vi "Main.vi"(8 "DB-Interface":refnum<class "DB-Interface.lvclass">, 9 "Call Chain":string[](array[string]), 10 "Config Section":string, 11 "Module Admin":refnum<class "Delacor_lib_QMH_Cloneable Module Admin.lvclass">) -> ()   [LabVIEW 2022 SP3, in "hse-db.lvlib" / "DB_CONNECTOR.lvlib"]
doc: "Database Connector DQMH module. \n\nThis module is a singleton. Every module or component within an application that needs database connectivity should load its own instance of this module and keep the reference private.\n\n____\nHAMPEL SOFTWARE ENGINEERING v1.4.0 (2023-12-19 09:52)"
uses:
  DB_CONNECTOR.lvlib
  <vilib>/Delacor/Delacor QMH/Libraries/Cloneable Module Admin_class/Delacor_lib_QMH_Cloneable Module Admin.lvclass
  C:/Program Files/National Instruments/LabVIEW 2022/vi.lib/Delacor/Delacor QMH/Libraries/Module Admin_class/Delacor_lib_QMH_Module Admin.lvclass
  DB-Interface/DB-Interface.lvclass
  Module Data--cluster.ctl
  hse-libraries/Source/hse-configuration/config-base/config-base.lvclass
  Stop Argument--cluster.ctl
  <vilib>/Delacor/Delacor QMH/Libraries/Message Queue_class/Delacor_lib_QMH_Message Queue.lvclass/Delacor_lib_QMH_Message Queue.ctl
  <vilib>/Delacor/Delacor QMH/Libraries/Module Admin_class/Delacor_lib_QMH_Module Admin.lvclass/Delacor_lib_QMH_Module Admin.ctl
  <vilib>/Delacor/Delacor QMH/Libraries/Cloneable Module Admin_class/Delacor_lib_QMH_Cloneable Module Admin.lvclass/Delacor_lib_QMH_Cloneable Module Admin.ctl
  Configure Argument--cluster.ctl
  Connect Argument--cluster.ctl
  Fast Query Argument--cluster.ctl
  Close Connection Argument--cluster.ctl
  Start Transaction Argument--cluster.ctl
  Get DB-Type Argument--cluster.ctl
  Get DB-Type (Reply Payload)--cluster.ctl
  Query Argument--cluster.ctl
  Query (Reply Payload)--cluster.ctl
  Commit Transaction Argument--cluster.ctl
  Commit Transaction (Reply Payload)--cluster.ctl
  Set Module Timeout Argument--cluster.ctl
  Rollback Transaction Argument--cluster.ctl
  Rollback Transaction (Reply Payload)--cluster.ctl
  Sub-VIs/timeout-fgv-actions--control.ctl
  <vilib>/Utility/miscctls.llb/LVPointTypeDef.ctl
  <vilib>/Delacor/Delacor QMH/Libraries/Message Queue_class/Delacor_lib_QMH_Enqueue Message (Single).vi
  <vilib>/Delacor/Delacor QMH/Libraries/Cloneable Module Admin_class/Delacor_lib_QMH_Get Module ID.vi
  <vilib>/Delacor/Delacor QMH/Libraries/Module Admin_class/Delacor_lib_QMH_Get External Launch.vi
  <vilib>/Utility/error.llb/Error Cluster From Error Code.vi
  <vilib>/ErrorRing/Error Ring.xnode
  <vilib>/Delacor/Delacor QMH/Libraries/Message Queue_class/Delacor_lib_QMH_Message Queue.lvclass
panel:
  out "Module Name":string
  out "error out":errorcluster
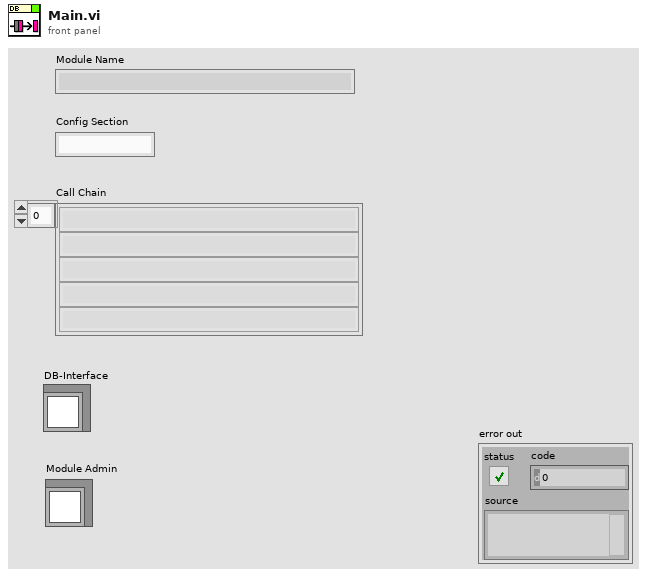
[diagram p1: front panel]
types:
  T1 = typedef "hse-db.lvlib/DB_CONNECTOR.lvlib/Request Events--cluster.ctl" = cluster{"Stop Module":refnum<user-event>, "Show Panel":refnum<user-event>, "Hide Panel":refnum<user-event>, "Show Diagram":refnum<user-event>, "Get Module Execution Status":refnum<user-event>, "Configure":refnum<user-event>, "Connect":refnum<user-event>, "Close Connection":refnum<user-event>, "Start Transaction":refnum<user-event>, "Fast Query":refnum<user-event>, "Get DB-Type":refnum<user-event>, "Query":refnum<user-event>, "Commit Transaction":refnum<user-event>, "Set Module Timeout":refnum<user-event>, "Rollback Transaction":refnum<user-event>}
  T2 = typedef "hse-db.lvlib/DB_CONNECTOR.lvlib/Module Data--cluster.ctl" = cluster{"hse-config":refnum<class "config-base.lvclass">, "Config Section":string, "DB-Interface":refnum<class "DB-Interface.lvclass">}
  T3 = enum32{"invalid lock state", "Not Locked", "Locked (No Password)", "Password-protected"}
  T4 = typedef "hse-db.lvlib/DB_CONNECTOR.lvlib/Stop Argument--cluster.ctl" = cluster{"Origin":string, "Module ID":i32, "Exit via Stop Module Req?":bool, "Wait for Module to stop?":bool}
  T5 = typedef "hse-db.lvlib/DB_CONNECTOR.lvlib/Configure Argument--cluster.ctl" = cluster{"Module ID":i32, "Boolean":bool}
  T6 = typedef "hse-db.lvlib/DB_CONNECTOR.lvlib/Connect Argument--cluster.ctl" = cluster{"Module ID":i32, "Boolean":bool}
  T7 = typedef "hse-db.lvlib/DB_CONNECTOR.lvlib/Fast Query Argument--cluster.ctl" = cluster{"Module ID":i32, "Query":string}
  T8 = typedef "hse-db.lvlib/DB_CONNECTOR.lvlib/Close Connection Argument--cluster.ctl" = cluster{"Module ID":i32, "Boolean":bool}
  T9 = typedef "hse-db.lvlib/DB_CONNECTOR.lvlib/Start Transaction Argument--cluster.ctl" = cluster{"Module ID":i32, "Boolean":bool}
  T10 = typedef "hse-db.lvlib/DB_CONNECTOR.lvlib/Get DB-Type Argument--cluster.ctl" = cluster{"Module ID":i32, "Wait Notifier":refnum<notifier>, "wait for reply":bool}
  T11 = typedef "hse-db.lvlib/DB_CONNECTOR.lvlib/Query Argument--cluster.ctl" = cluster{"Module ID":i32, "Query":string, "Wait Notifier":refnum<notifier>, "wait for reply":bool}
  T12 = typedef "hse-db.lvlib/DB_CONNECTOR.lvlib/Commit Transaction Argument--cluster.ctl" = cluster{"Module ID":i32, "Wait Notifier":refnum<notifier>, "wait for reply":bool}
  T13 = typedef "hse-db.lvlib/DB_CONNECTOR.lvlib/Set Module Timeout Argument--cluster.ctl" = cluster{"Module ID":i32, "Module Timeout":i32}
  T14 = typedef "hse-db.lvlib/DB_CONNECTOR.lvlib/Rollback Transaction Argument--cluster.ctl" = cluster{"Module ID":i32, "Wait Notifier":refnum<notifier>, "wait for reply":bool}
  T15 = typedef "hse-db.lvlib/DB_CONNECTOR.lvlib/timeout-fgv-actions--control.ctl" = enum16{"set", "get"}
  T16 = typedef "LVPointTypeDef.ctl" = cluster{"Horizontal":i16, "Vertical":i16}
  T17 = enum32{"Invalid", "Standard", "Closed", "Hidden", "Minimized", "Maximized"}
  T18 = typedef "hse-db.lvlib/DB_CONNECTOR.lvlib/Query (Reply Payload)--cluster.ctl" = cluster{"Return Data":string[][], "Meta Data":variant, "Field Names":string[], "Query_error":errorcluster, "Module ID":i32}
  T19 = typedef "hse-db.lvlib/DB_CONNECTOR.lvlib/Commit Transaction (Reply Payload)--cluster.ctl" = cluster{"Commit Transaction_error":errorcluster, "Module ID":i32}
  T20 = typedef "hse-db.lvlib/DB_CONNECTOR.lvlib/Rollback Transaction (Reply Payload)--cluster.ctl" = cluster{"Rollback Transaction_error":errorcluster, "Module ID":i32}
  T21 = typedef "hse-db.lvlib/DB_CONNECTOR.lvlib/Get DB-Type (Reply Payload)--cluster.ctl" = cluster{"DB-Type":string, "error":errorcluster, "Module ID":i32}
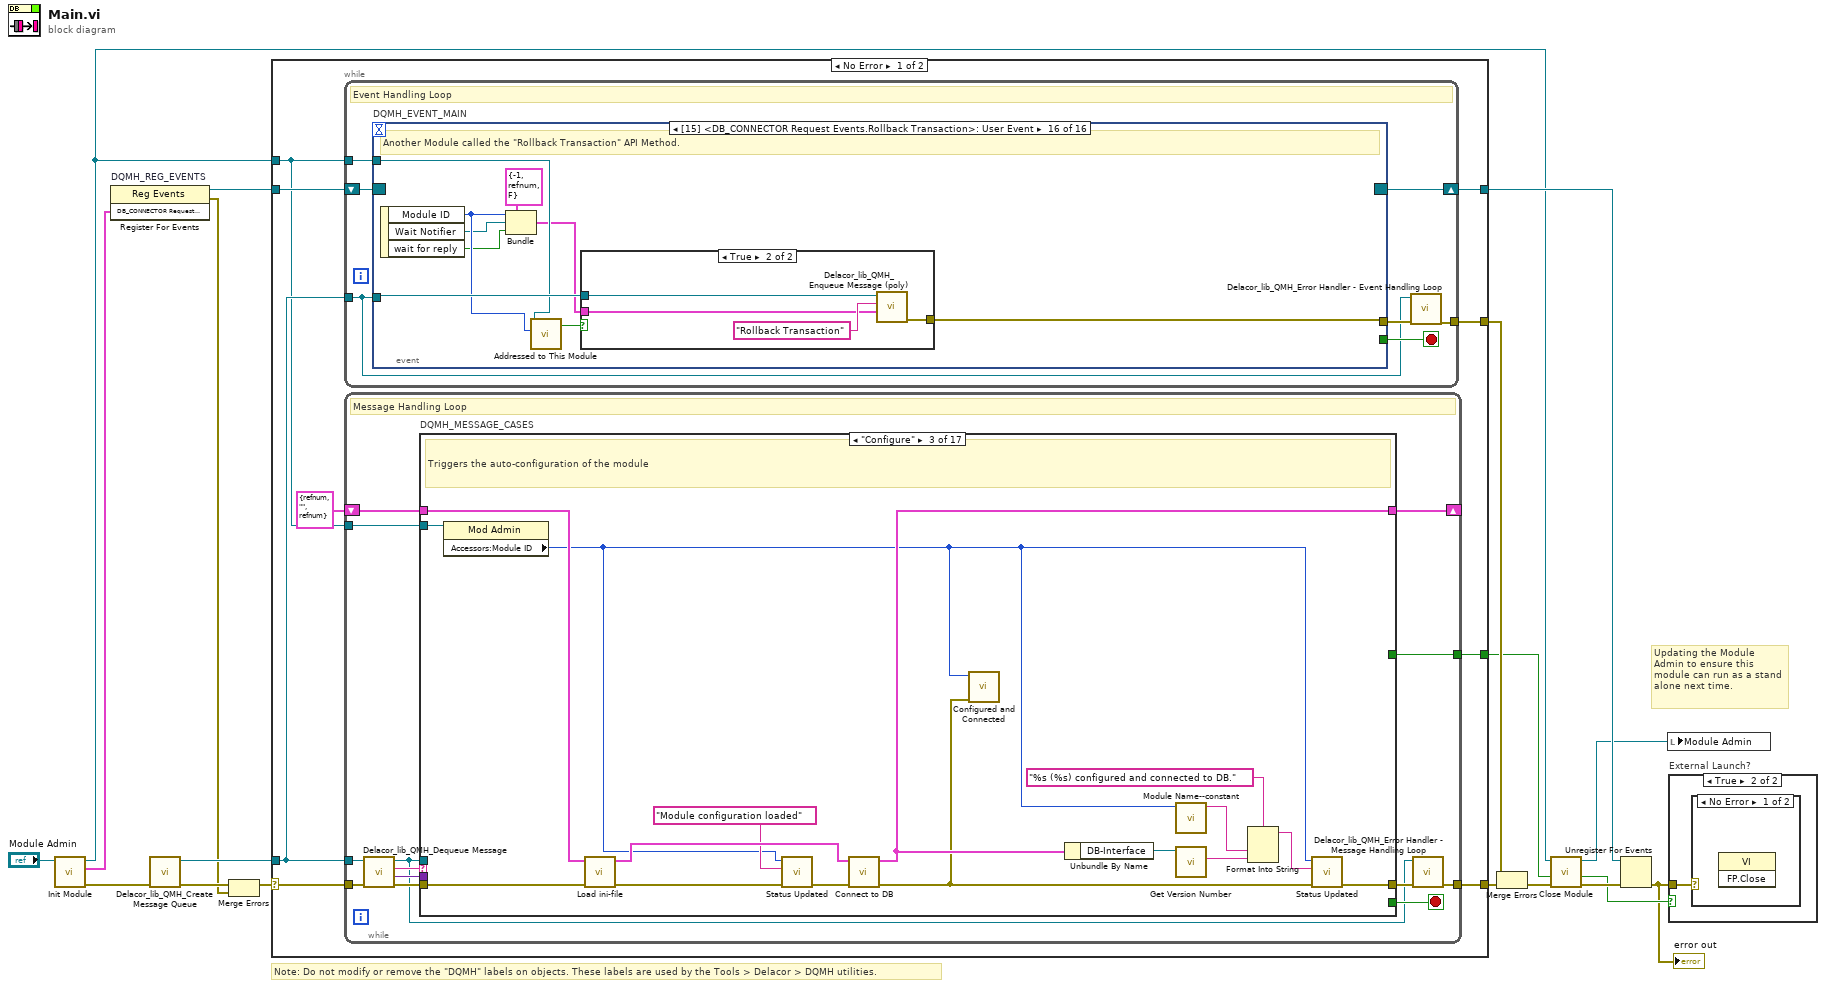
[diagram p0: block diagram]
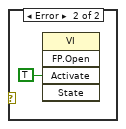
[diagram p3: hidden frame]
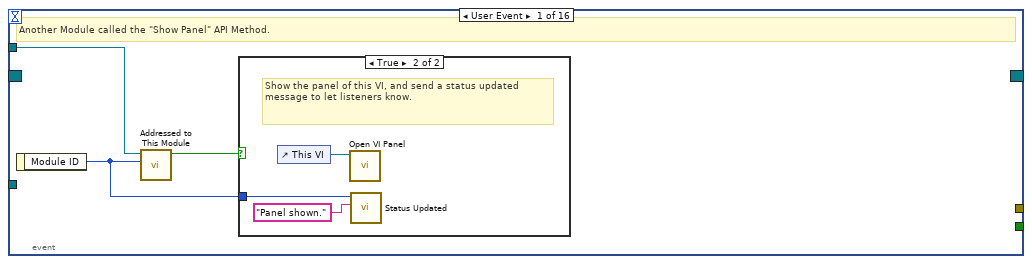
[diagram p4: hidden frame]
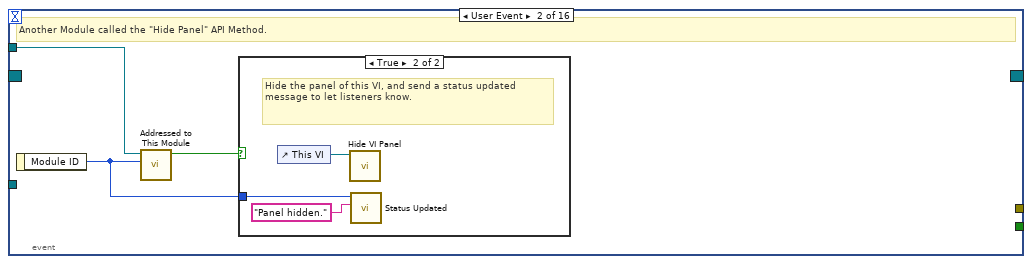
[diagram p6: hidden frame]
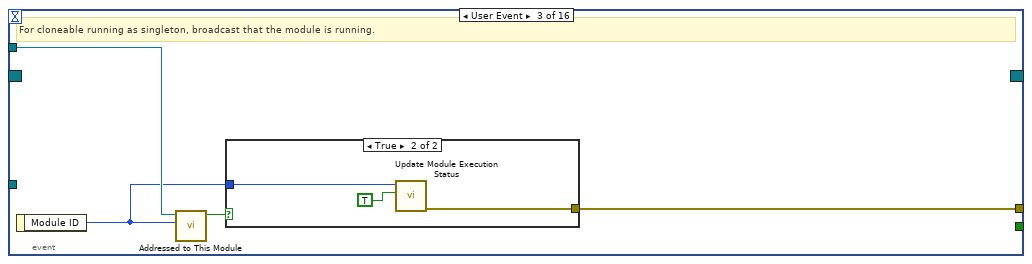
[diagram p8: hidden frame]
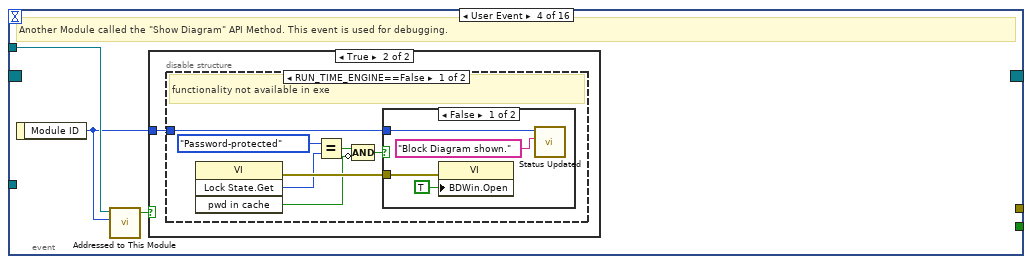
[diagram p10: hidden frame]
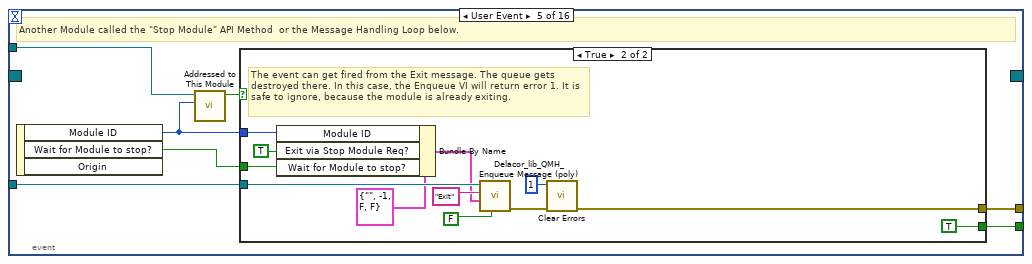
[diagram p14: hidden frame]
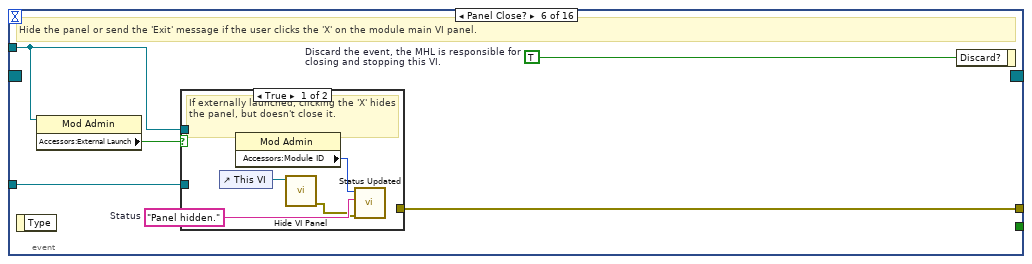
[diagram p16: hidden frame]
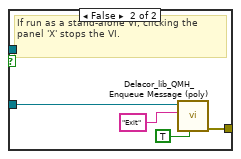
[diagram p17: hidden frame]
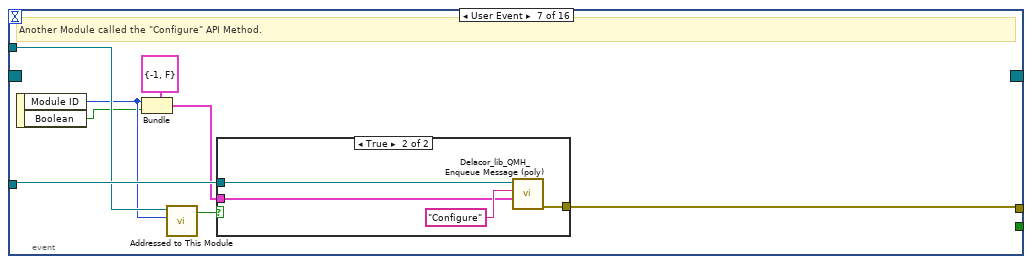
[diagram p18: hidden frame]
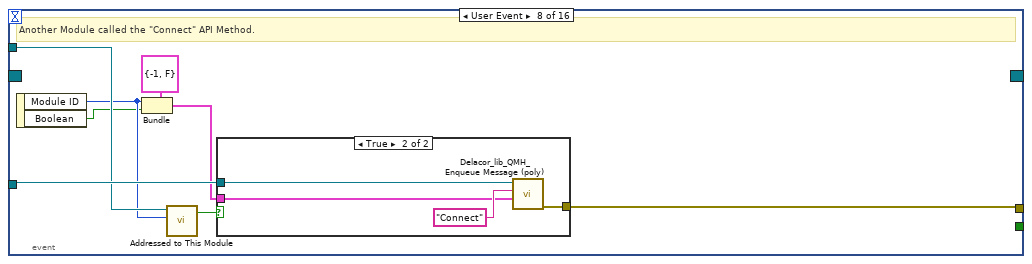
[diagram p20: hidden frame]
diagram:
  # "Note: Do not modify or remove the \"DQMH\" labels on objects. These labels are used by the Tools > Delacor > DQMH utilities."
  # "Updating the Module Admin to ensure this module can run as a stand alone next time."
  n1 = call "Init Module.vi"("Cloneable Module Admin in"="Module Admin") -> ("error out"=w15:errorcluster, "DB_CONNECTOR Request Events"=w12:T1, "Cloneable Module Admin out"=w8:refnum<class "Delacor_lib_QMH_Cloneable Module Admin.lvclass">)  [unwired: 8 in]
  n2 = register-events "DQMH_REG_EVENTS"(w12) -> (reference out=w13:refnum<event-registration>, error out=w3:errorcluster)  [unwired: 2 in]
  n3 = call <vilib>:"Delacor_lib_QMH_Create Message Queue.vi"("error in"=w15) -> ("error out"=w5:errorcluster, "Message Queue"=w11:refnum<class "Delacor_lib_QMH_Message Queue.lvclass">)  [unwired: 9 in]
  n4 = Merge Errors(w5, w3) -> (w4:errorcluster)
  n5 = case shown="No Error" w4 {
    selector: w4 -> [w21 w514]
    tunnel: [w27 w514] -> w16
    tunnel: [w26 w515] -> w14
    tunnel: w13 -> [w24 w515]
    tunnel: w11 -> [w23 w507]
    tunnel: [w22 _] -> w17
    tunnel: w8 -> [w20 w510]
    tunnel: [w19 _] -> w7
    frame No Error {
      n6 = while {
        tunnel: w23 -> [w28]
        shift-right: [w33] -> w26
        shift-left: w24 -> [w34]
        tunnel: [w30] -> w22
        tunnel: w20 -> [w29]
        stop <- w31 stop-if-true
        # "Event Handling Loop"
        n7 = event "DQMH_EVENT_MAIN" shown="[15] <DB_CONNECTOR Request Events.Rollback Transaction>: User Event" {
          selector: w34 -> [_ _ _ _ _ _ _ _ _ _ _ _ _ _ _ _]
          dyn-events: [_ _ _ _ _ _ _ _ _ _ _ _ _ _ _ _] -> w33
          timeout: _ -> [_ _ _ _ _ _ _ _ _ _ _ _ _ _ _ _]
          tunnel: [_ _ _ _ w72 _ _ _ _ _ _ _ _ _ _ _] -> w31
          tunnel: w28 -> [_ _ _ _ w75 w91 w109 w121 w133 w145 w157 w170 w184 w197 w209 w222]
          tunnel: [_ _ w48 _ w69 w89 w102 w114 w126 w138 w150 w162 w179 w192 w202 w214] -> w32
          tunnel: w29 -> [w36 w42 w49 w55 w74 w88 w107 w119 w131 w143 w155 w168 w182 w195 w207 w220]
          event User Event {
            # "Another Module called the \"Show Panel\" API Method."
            n8 = event-data() -> ("Module ID"=w35:i32)  [unwired: 1 in]
            n9 = call "Addressed to This Module.vi"("Module ID from Argument"=w35, "Module Admin"=w36) -> ("Addressed to this instance?"=w37:bool)  [unwired: 8 in, 1 out]
            n10 = case shown="True" w37 {
              tunnel: w35 -> [_ w38]
              frame False {
              }
              frame True {
                # "Show the panel of this VI, and send a status updated message to let listeners know."
                n11 = control-ref of="This VI"() -> (w40:refnum<vi>)
                n12 = call "Open VI Panel.vi"("VI"=w40) -> ()  [unwired: 10 in, 1 out]
                n13 = call "Status Updated.vi"("Status"="Panel shown." ("format string"), "Module ID"=w38) -> ()  [unwired: 9 in, 1 out]
              }
            }
          }
          event User Event {
            # "Another Module called the \"Hide Panel\" API Method."
            n14 = event-data() -> ("Module ID"=w41:i32)  [unwired: 1 in]
            n15 = call "Addressed to This Module.vi"("Module ID from Argument"=w41, "Module Admin"=w42) -> ("Addressed to this instance?"=w43:bool)  [unwired: 8 in, 1 out]
            n16 = case shown="True" w43 {
              tunnel: w41 -> [_ w44]
              frame False {
              }
              frame True {
                # "Hide the panel of this VI, and send a status updated message to let listeners know."
                n17 = control-ref of="This VI"() -> (w46:refnum<vi>)
                n18 = call "Hide VI Panel.vi"("VI"=w46) -> ()  [unwired: 10 in, 1 out]
                n19 = call "Status Updated.vi"("Status"="Panel hidden." ("format string"), "Module ID"=w44) -> ()  [unwired: 9 in, 1 out]
              }
            }
          }
          event User Event {
            # "For cloneable running as singleton, broadcast that the module is running."
            n20 = event-data() -> ("Module ID"=w47:i32)  [unwired: 1 in]
            n21 = call "Addressed to This Module.vi"("Module ID from Argument"=w47, "Module Admin"=w49) -> ("Addressed to this instance?"=w50:bool)  [unwired: 8 in, 1 out]
            n22 = case shown="True" w50 {
              tunnel: [_ w53] -> w48
              tunnel: w47 -> [_ w52]
              frame False {
              }
              frame True {
                n23 = call "Update Module Execution Status.vi"("Running?"=TRUE, "Module ID"=w52) -> ("error out"=w53:errorcluster)  [unwired: 9 in]
              }
            }
          }
          event User Event {
            # "Another Module called the \"Show Diagram\" API Method. This event is used for debugging."
            n24 = event-data() -> ("Module ID"=w54:i32)  [unwired: 1 in]
            n25 = call "Addressed to This Module.vi"("Module ID from Argument"=w54, "Module Admin"=w55) -> ("Addressed to this instance?"=w56:bool)  [unwired: 8 in, 1 out]
            n26 = case shown="True" w56 {
              tunnel: w54 -> [_ w57]
              frame False {
              }
              frame True {
                n27 = disable-structure shown="RUN_TIME_ENGINE==False" {
                  disable-tunnel: w57 -> [w58 _]
                  frame condition #0 (active) {
                    # "functionality not available in exe"
                    n28 = invoke on="Invoke Node" class="VI" method="Lock State.Get"() -> (error out=w64:errorcluster, "Get Lock State"=w63:T3, "pwd in cache"=w60:bool)  [unwired: 4 in, 1 out]
                    n29 = Equal?(x=T3."Password-protected", y=w63) -> (x = y?=w61:bool)
                    n30 = Compound Arithmetic op=AND(w61, invert w60) -> (w59:bool)
                    n31 = case shown="False" w59 {
                      tunnel: w64 -> [w67 _]
                      tunnel: w58 -> [w65 _]
                      frame False {
                        n32 = property on="Property Node" class="VI"(error in=w67, "BDWin.Open"=TRUE ("Block Diagram Window:Open")) -> ()  [unwired: 1 in, 2 out]
                        n33 = call "Status Updated.vi"("Status"="Block Diagram shown." ("format string"), "Module ID"=w65) -> ()  [unwired: 9 in, 1 out]
                      }
                      frame True {
                        # "Password-protected VI, and the password is not in the cache. Do not show the diagram."
                      }
                    }
                  }
                  frame condition #1 {
                  }
                }
              }
            }
          }
          event User Event {
            # "Another Module called the \"Stop Module\" API Method  or the Message Handling Loop below."
            n34 = event-data() -> ("Module ID"=w70:i32, "Wait for Module to stop?"=w71:bool)  [unwired: 1 in, 1 out]
            n35 = call "Addressed to This Module.vi"("Module ID from Argument"=w70, "Module Admin"=w74) -> ("Addressed to this instance?"=w73:bool)  [unwired: 8 in, 1 out]
            n36 = case shown="True" w73 {
              tunnel: [_ w77] -> w69
              tunnel: w75 -> [_ w83]
              tunnel: [_ TRUE] -> w72
              tunnel: w71 -> [_ w79]
              tunnel: w70 -> [_ w76]
              frame False {
              }
              frame True {
                # "The event can get fired from the Exit message. The queue gets destroyed there. In this case, the Enqueue VI will return error 1. It is safe to ignore, because the module is already exiting."
                n37 = Bundle By Name(cluster=T4 {"Origin"="", "Module ID"=-1, "Exit via Stop Module Req?"=FALSE, "Wait for Module to stop?"=FALSE} ("Stop Argument"), "Module ID"=w76, "Exit via Stop Module Req?"=TRUE, "Wait for Module to stop?"=w79) -> (w78:T4)
                n38 = call-poly <vilib>:"Delacor_lib_QMH_Enqueue Message (poly).vi"("Priority Message? (F)"=FALSE, "Message Data"=w78, "Message"="Exit", "Message Queue in"=w83) -> ("error out"=w86:errorcluster)  [unwired: 6 in, 1 out]
                n39 = call <vilib>:"Clear Errors.vi"("error in (no error)"=w86, "specific error code to clear (0: all)"=1) -> ("error out"=w77:errorcluster)  [unwired: 4 in, 1 out]
              }
            }
          }
          event Panel Close? {
            w92 = TRUE  # Discard the event, the MHL is responsible for closing and stopping this VI.
            # "Hide the panel or send the 'Exit' message if the user clicks the 'X' on the module main VI panel."
            n40 = event-data() -> ()  [unwired: 1 in, 1 out]
            n41 = property on="Property Node" class="Mod Admin"(reference=w88) -> ("Accessors:External Launch"=w90:bool)  [unwired: 1 in, 2 out]
            n42 = case shown="True" w90 {
              tunnel: w91 -> [_ w101]
              tunnel: [_ w100] -> w89
              tunnel: w88 -> [w95 _]
              frame True {
                w96 = "Panel hidden."  # Status
                # "If externally launched, clicking the 'X' hides the panel, but doesn't close it."
                n43 = control-ref of="This VI"() -> (w97:refnum<vi>)
                n44 = property class="Mod Admin"(reference=w95) -> ("Accessors:Module ID"=w94:i32)  [unwired: 1 in, 2 out]
                n45 = call "Hide VI Panel.vi"("VI"=w97) -> ("error out"=w93:errorcluster)  [unwired: 10 in]
                n46 = call "Status Updated.vi"("error in (no error)"=w93, "Status"=w96, "Module ID"=w94) -> ()  [unwired: 8 in, 1 out]
              }
              frame False {
                # "If run as a stand-alone VI, clicking the panel 'X' stops the VI."
                n47 = call-poly <vilib>:"Delacor_lib_QMH_Enqueue Message (poly).vi"("Priority Message? (F)"=TRUE, "Message"="Exit", "Message Queue in"=w101) -> ("error out"=w100:errorcluster)  [unwired: 7 in, 1 out]
              }
            }
            n48 = event-data ("Event Filter Node")("Discard?"=w92) -> ()  [unwired: 1 in, 1 out]
          }
          event User Event {
            # "Another Module called the \"Configure\" API Method."
            n49 = event-data() -> ("Module ID"=w104:i32, "Boolean"=w103:bool)  [unwired: 1 in]
            n50 = Bundle(cluster=T5 {"Module ID"=-1, "Boolean"=FALSE} ("Configure Argument"), "Module ID"=w104, "Boolean"=w103) -> (w105:T5)
            n51 = call "Addressed to This Module.vi"("Module ID from Argument"=w104, "Module Admin"=w107) -> ("Addressed to this instance?"=w108:bool)  [unwired: 8 in, 1 out]
            n52 = case shown="True" w108 {
              tunnel: w109 -> [_ w113]
              tunnel: w105 -> [_ w111]
              tunnel: [_ w110] -> w102
              frame False {
              }
              frame True {
                n53 = call-poly <vilib>:"Delacor_lib_QMH_Enqueue Message (poly).vi"("Message Data"=w111, "Message"="Configure", "Message Queue in"=w113) -> ("error out"=w110:errorcluster)  [unwired: 7 in, 1 out]
              }
            }
          }
          event User Event {
            # "Another Module called the \"Connect\" API Method."
            n54 = event-data() -> ("Module ID"=w116:i32, "Boolean"=w115:bool)  [unwired: 1 in]
            n55 = Bundle(cluster=T6 {"Module ID"=-1, "Boolean"=FALSE} ("Connect Argument"), "Module ID"=w116, "Boolean"=w115) -> (w117:T6)
            n56 = call "Addressed to This Module.vi"("Module ID from Argument"=w116, "Module Admin"=w119) -> ("Addressed to this instance?"=w120:bool)  [unwired: 8 in, 1 out]
            n57 = case shown="True" w120 {
              tunnel: w121 -> [_ w125]
              tunnel: w117 -> [_ w123]
              tunnel: [_ w122] -> w114
              frame False {
              }
              frame True {
                n58 = call-poly <vilib>:"Delacor_lib_QMH_Enqueue Message (poly).vi"("Message Data"=w123, "Message"="Connect", "Message Queue in"=w125) -> ("error out"=w122:errorcluster)  [unwired: 7 in, 1 out]
              }
            }
          }
          event User Event {
            # "Another Module called the \"Fast Query\" API Method."
            n59 = event-data() -> ("Module ID"=w128:i32, "Query"=w127:string)  [unwired: 1 in]
            n60 = Bundle(cluster=T7 {"Module ID"=-1, "Query"=""} ("Fast Query Argument"), "Module ID"=w128, "Query"=w127) -> (w129:T7)
            n61 = call "Addressed to This Module.vi"("Module ID from Argument"=w128, "Module Admin"=w131) -> ("Addressed to this instance?"=w132:bool)  [unwired: 8 in, 1 out]
            n62 = case shown="True" w132 {
              tunnel: w133 -> [_ w137]
              tunnel: w129 -> [_ w135]
              tunnel: [_ w134] -> w126
              frame False {
              }
              frame True {
                n63 = call-poly <vilib>:"Delacor_lib_QMH_Enqueue Message (poly).vi"("Message Data"=w135, "Message"="Fast Query", "Message Queue in"=w137) -> ("error out"=w134:errorcluster)  [unwired: 7 in, 1 out]
              }
            }
          }
          event User Event {
            # "Another Module called the \"Close Connection\" API Method."
            n64 = event-data() -> ("Module ID"=w140:i32, "Boolean"=w139:bool)  [unwired: 1 in]
            n65 = Bundle(cluster=T8 {"Module ID"=-1, "Boolean"=FALSE} ("Close Connection Argument"), "Module ID"=w140, "Boolean"=w139) -> (w141:T8)
            n66 = call "Addressed to This Module.vi"("Module ID from Argument"=w140, "Module Admin"=w143) -> ("Addressed to this instance?"=w144:bool)  [unwired: 8 in, 1 out]
            n67 = case shown="True" w144 {
              tunnel: w145 -> [_ w149]
              tunnel: w141 -> [_ w147]
              tunnel: [_ w146] -> w138
              frame False {
              }
              frame True {
                n68 = call-poly <vilib>:"Delacor_lib_QMH_Enqueue Message (poly).vi"("Message Data"=w147, "Message"="Close Connection", "Message Queue in"=w149) -> ("error out"=w146:errorcluster)  [unwired: 7 in, 1 out]
              }
            }
          }
          event User Event {
            # "Another Module called the \"Start Transaction\" API Method."
            n69 = event-data() -> ("Module ID"=w152:i32, "Boolean"=w151:bool)  [unwired: 1 in]
            n70 = Bundle(cluster=T9 {"Module ID"=-1, "Boolean"=FALSE} ("Start Transaction Argument"), "Module ID"=w152, "Boolean"=w151) -> (w153:T9)
            n71 = call "Addressed to This Module.vi"("Module ID from Argument"=w152, "Module Admin"=w155) -> ("Addressed to this instance?"=w156:bool)  [unwired: 8 in, 1 out]
            n72 = case shown="True" w156 {
              tunnel: w157 -> [_ w161]
              tunnel: w153 -> [_ w159]
              tunnel: [_ w158] -> w150
              frame False {
              }
              frame True {
                n73 = call-poly <vilib>:"Delacor_lib_QMH_Enqueue Message (poly).vi"("Message Data"=w159, "Message"="Start Transaction", "Message Queue in"=w161) -> ("error out"=w158:errorcluster)  [unwired: 7 in, 1 out]
              }
            }
          }
          event User Event {
            # "Another Module called the \"Get DB-Type\" API Method."
            n74 = event-data() -> ("Module ID"=w165:i32, "Wait Notifier"=w164:refnum<notifier>, "wait for reply"=w163:bool)  [unwired: 1 in]
            n75 = Bundle(cluster=T10 {"Module ID"=-1, "Wait Notifier"=refnum, "wait for reply"=FALSE} ("Get DB-Type Argument"), "Module ID"=w165, "Wait Notifier"=w164, "wait for reply"=w163) -> (w166:T10)
            n76 = call "Addressed to This Module.vi"("Module ID from Argument"=w165, "Module Admin"=w168) -> ("Addressed to this instance?"=w169:bool)  [unwired: 8 in, 1 out]
            n77 = case shown="True" w169 {
              tunnel: w170 -> [_ w174]
              tunnel: w166 -> [_ w172]
              tunnel: [_ w171] -> w162
              frame False {
              }
              frame True {
                n78 = call-poly <vilib>:"Delacor_lib_QMH_Enqueue Message (poly).vi"("Message Data"=w172, "Message"="Get DB-Type", "Message Queue in"=w174) -> ("error out"=w171:errorcluster)  [unwired: 7 in, 1 out]
              }
            }
          }
          event User Event {
            # "Another Module called the \"Query\" API Method."
            n79 = event-data() -> ("Module ID"=w175:i32, "Query"=w178:string, "Wait Notifier"=w177:refnum<notifier>, "wait for reply"=w176:bool)  [unwired: 1 in]
            n80 = Bundle(cluster=T11 {"Module ID"=-1, "Query"="", "Wait Notifier"=refnum, "wait for reply"=FALSE} ("Query Argument"), "Module ID"=w175, "Query"=w178, "Wait Notifier"=w177, "wait for reply"=w176) -> (w180:T11)
            n81 = call "Addressed to This Module.vi"("Module ID from Argument"=w175, "Module Admin"=w182) -> ("Addressed to this instance?"=w183:bool)  [unwired: 8 in, 1 out]
            n82 = case shown="True" w183 {
              tunnel: w184 -> [_ w188]
              tunnel: w180 -> [_ w186]
              tunnel: [_ w185] -> w179
              frame False {
              }
              frame True {
                n83 = call-poly <vilib>:"Delacor_lib_QMH_Enqueue Message (poly).vi"("Message Data"=w186, "Message"="Query", "Message Queue in"=w188) -> ("error out"=w185:errorcluster)  [unwired: 7 in, 1 out]
              }
            }
          }
          event User Event {
            # "Another Module called the \"Commit Transaction\" API Method."
            n84 = event-data() -> ("Module ID"=w189:i32, "Wait Notifier"=w191:refnum<notifier>, "wait for reply"=w190:bool)  [unwired: 1 in]
            n85 = Bundle(cluster=T12 {"Module ID"=-1, "Wait Notifier"=refnum, "wait for reply"=FALSE} ("Commit Transaction Argument"), "Module ID"=w189, "Wait Notifier"=w191, "wait for reply"=w190) -> (w193:T12)
            n86 = call "Addressed to This Module.vi"("Module ID from Argument"=w189, "Module Admin"=w195) -> ("Addressed to this instance?"=w196:bool)  [unwired: 8 in, 1 out]
            n87 = case shown="True" w196 {
              tunnel: w197 -> [_ w201]
              tunnel: w193 -> [_ w199]
              tunnel: [_ w198] -> w192
              frame False {
              }
              frame True {
                n88 = call-poly <vilib>:"Delacor_lib_QMH_Enqueue Message (poly).vi"("Message Data"=w199, "Message"="Commit Transaction", "Message Queue in"=w201) -> ("error out"=w198:errorcluster)  [unwired: 7 in, 1 out]
              }
            }
          }
          event User Event {
            # "Another Module called the \"Set Module Timeout\" API Method."
            n89 = event-data() -> ("Module ID"=w204:i32, "Module Timeout"=w203:i32)  [unwired: 1 in]
            n90 = Bundle(cluster=T13 {"Module ID"=-1, "Module Timeout"=0} ("Set Module Timeout Argument"), "Module ID"=w204, "Module Timeout"=w203) -> (w205:T13)
            n91 = call "Addressed to This Module.vi"("Module ID from Argument"=w204, "Module Admin"=w207) -> ("Addressed to this instance?"=w208:bool)  [unwired: 8 in, 1 out]
            n92 = case shown="True" w208 {
              tunnel: w209 -> [_ w213]
              tunnel: w205 -> [_ w211]
              tunnel: [_ w210] -> w202
              frame False {
              }
              frame True {
                n93 = call-poly <vilib>:"Delacor_lib_QMH_Enqueue Message (poly).vi"("Message Data"=w211, "Message"="Set Module Timeout", "Message Queue in"=w213) -> ("error out"=w210:errorcluster)  [unwired: 7 in, 1 out]
              }
            }
          }
          event User Event {
            # "Another Module called the \"Rollback Transaction\" API Method."
            n94 = event-data() -> ("Module ID"=w217:i32, "Wait Notifier"=w216:refnum<notifier>, "wait for reply"=w215:bool)  [unwired: 1 in]
            n95 = Bundle(cluster=T14 {"Module ID"=-1, "Wait Notifier"=refnum, "wait for reply"=FALSE} ("Rollback Transaction Argument"), "Module ID"=w217, "Wait Notifier"=w216, "wait for reply"=w215) -> (w218:T14)
            n96 = call "Addressed to This Module.vi"("Module ID from Argument"=w217, "Module Admin"=w220) -> ("Addressed to this instance?"=w221:bool)  [unwired: 8 in, 1 out]
            n97 = case shown="True" w221 {
              tunnel: w222 -> [_ w226]
              tunnel: w218 -> [_ w224]
              tunnel: [_ w223] -> w214
              frame False {
              }
              frame True {
                n98 = call-poly <vilib>:"Delacor_lib_QMH_Enqueue Message (poly).vi"("Message Data"=w224, "Message"="Rollback Transaction", "Message Queue in"=w226) -> ("error out"=w223:errorcluster)  [unwired: 7 in, 1 out]
              }
            }
          }
        }
        n99 = call-dynamic "Delacor_lib_QMH_Error Handler - Event Handling Loop.vi"("error in"=w32, "Message Queue in"=w28) -> ("dup error in"=w30:errorcluster)  [unwired: 8 in, 1 out]
      }
      n100 = while {
        tunnel: w23 -> [w231]
        shift-right: [w237] -> _
        shift-left: T2 {"hse-config"=refnum, "Config Section"="", "DB-Interface"=refnum} ("Data Cluster") -> [w238]
        tunnel: w21 -> [w235]
        tunnel: [w229] -> w27
        tunnel: w20 -> [w228]
        tunnel: [w227] -> w19
        stop <- w236 stop-if-true
        # "Message Handling Loop"
        n101 = call-dynamic "Delacor_lib_QMH_Dequeue Message.vi"("error in"=w235, "Message Queue in"=w231) -> ("error out"=w234:errorcluster, "Message Data"=w232:variant, "Message"=w233:string, "Message Queue out"=w230:refnum<class "Delacor_lib_QMH_Message Queue.lvclass">)  [unwired: 6 in]
        n102 = case "DQMH_MESSAGE_CASES" shown="\"Configure\"" w233 {
          selector: w233 -> [_ _ _ _ _ _ _ _ _ _ _ _ _ _ _ _ w496]
          tunnel: w230 -> [_ _ _ _ _ _ _ _ _ _ _ _ _ _ w456 w476 _]
          tunnel: w234 -> [w263 w278 w294 w302 w322 w355 w360 w375 w400 w412 w425 w444 w452 w454 w465 w490 w491]
          tunnel: [w247 w278 w286 w297 w316 w339 w356 w369 w392 w406 w424 w436 w450 w454 w455 w479 w492] -> w239
          tunnel: w238 -> [w250 w277 w293 w301 w314 w343 w359 w367 w391 w411 w418 w443 w451 w453 w464 w474 w498]
          tunnel: [w249 w277 w281 w300 w313 w342 w358 w366 w389 w410 w418 w443 w451 w453 w464 w473 w498] -> w237
          tunnel: [_ _ _ _ _ _ _ _ _ _ _ _ _ _ _ w489 _] -> w236
          tunnel: w232 -> [_ _ _ _ w321 w353 _ w374 w399 _ w423 w442 _ _ w463 w485 _]
          tunnel: w228 -> [w259 _ w292 w299 w306 w341 _ w362 w385 w407 w414 _ _ _ w460 w481 w494]
          tunnel: [_ _ _ _ _ _ _ _ _ _ _ _ _ _ _ w483 _] -> w227
          frame "Initialize" {
            # "Initialize - Any operation that needs to be done before the module can receive messages. Synchronize Caller Events.vi will inform Start Module.vi that the module has launched and is ready to receive messages. Module Did Init.vi will broadcast that the module initialized."
            n103 = call "Synchronize Caller Events.vi"("error in (no error)"=w263, "Module Admin"=w259) -> ("error out"=w261:errorcluster, "Module Admin out"=w258:refnum<class "Delacor_lib_QMH_Cloneable Module Admin.lvclass">)  [unwired: 8 in]
            n104 = property on="Property Node" class="Mod Admin"(reference=w258) -> ("Accessors:Module ID"=w240:i32, "Accessors:External Launch"=w260:bool)  [unwired: 1 in, 2 out]
            n105 = call <vilib>:"Get LV Class Name.vi"("object"="DB-Interface") -> ("class name"=w243:string)  [unwired: 9 in, 1 out]
            n106 = call "Module Name--constant.vi"("Module ID"=w240) -> ("Module Name"=w264:string)  [unwired: 10 in]
            "Module Name" <- w264
            n107 = call "Module Name--constant.vi"("Module ID"=w240) -> ("Module Name"=w257:string)  [unwired: 10 in]
            n108 = Bundle By Name(cluster=w250, "Config Section"="Config Section", "DB-Interface"="DB-Interface") -> (w249:T2)
            n109 = disable-structure shown="TARGET_TYPE==Windows||EMBEDDED_UI==TRUE" {
              disable-tunnel: w264 -> [w272 _]
              disable-tunnel: w260 -> [w268 _]
              frame condition #0 (active) {
                n110 = property on="Property Node" class="VI"("Front Panel.Title"=w272) -> (reference out=w275:refnum<vi>, error out=w276:errorcluster)  [unwired: 2 in]
                n111 = Select(t=T17."Hidden" ("State"), s=w268, f=T17."Standard" ("State")) -> (s? t:f=w269:T17)
                n112 = invoke on="Invoke Node" class="VI" method="FP.Open"(reference=w275, error in=w276, "State"=w269) -> (reference out=w274:refnum<vi>, error out=w273:errorcluster)  [unwired: 2 in, 3 out]
                n113 = invoke on="Invoke Node" class="VI" method="FP.Center"(reference=w274, error in=w273) -> ()  [unwired: 1 in, 3 out]
                n114 = property on="Pane" class="Pane"("Origin"=T16 {"Horizontal"=0, "Vertical"=0}) -> ()  [unwired: 2 in, 2 out]
              }
              frame condition #1 {
              }
            }
            n115 = call "Module Did Init.vi"("error in (no error)"=w261, "Initialized?"=TRUE, "Origin"=w257, "Module ID"=w240) -> ("error out"=w248:errorcluster)  [unwired: 7 in]
            n116 = case "Called with abstract parent?" shown="\"hse-db.lvlib:DB-Interface.lvclass\"" w243 {
              tunnel: w240 -> [_ w265]
              frame Default {
                # "no - everything okay"
              }
              frame "hse-db.lvlib:DB-Interface.lvclass" {
                # "yes - throw error"
                n117 = call "Status Updated.vi"("Status"="DB_Connector was initialized with DB-Interface.lvclass. Use a DB-Engine instead." ("class name"), "Module ID"=w265) -> ()  [unwired: 9 in, 1 out]
              }
            }
            n118 = Reverse 1D Array(array="Call Chain") -> (reversed array=w254:string[])
            n119 = Index Array(array=w254) -> (element=w253:string)  [unwired: 1 in]
            n120 = Match Pattern(string=w253, regular expression=".lvlib") -> (before substring=w251:string)  [unwired: 1 in, 3 out]
            n121 = Format Into String(format string="%s initialised from %s", w257, w251) -> (resulting string=w246:string)  [unwired: 2 in, 1 out]
            n122 = call "Status Updated.vi"("error in (no error)"=w248, "Status"=w246, "Module ID"=w240) -> ("error out"=w247:errorcluster)  [unwired: 8 in]
            n123 = call "timeout--fgv.vi"("Module ID"=w240, "Action"=timeout-fgv-actions--control."set", "Module Timeout in"=5000) -> ()  [unwired: 8 in, 1 out]
          }
          frame "--- Module Specific ---" {
            # "Separator -- The following cases handle messages specific to this Module."
          }
          frame "Configure" {
            # "Triggers the auto-configuration of the module"
            n124 = property on="Property Node" class="Mod Admin"(reference=w292) -> ("Accessors:Module ID"=w279:i32)  [unwired: 1 in, 2 out]
            n125 = call "Load ini-file.vi"("error in"=w294, "Data Cluster in"=w293) -> ("error out"=w291:errorcluster, "Data Cluster out"=w289:T2)  [unwired: 8 in]
            n126 = call "Status Updated.vi"("error in (no error)"=w291, "Status"="Module configuration loaded", "Module ID"=w279) -> ("error out"=w290:errorcluster)  [unwired: 8 in]
            n127 = call "Connect to DB.vi"("error in"=w290, "Data Cluster in"=w289) -> ("error out"=w280:errorcluster, "Data Cluster out"=w281:T2)  [unwired: 8 in]
            n128 = call "Configured and Connected.vi"("error in"=w280, "Module ID"=w279) -> ()  [unwired: 9 in, 1 out]
            n129 = Unbundle By Name(w281) -> ("DB-Interface"=w283:refnum<class "DB-Interface.lvclass">)
            n130 = call "Module Name--constant.vi"("Module ID"=w279) -> ("Module Name"=w288:string)  [unwired: 10 in]
            n131 = call-dynamic "Get Version Number.vi"("DB-Interface in"=w283) -> ("Version Number"=w282:string)  [unwired: 8 in, 2 out]
            n132 = Format Into String(format string="%s (%s) configured and connected to DB.", w288, w282) -> (resulting string=w285:string)  [unwired: 2 in, 1 out]
            n133 = call "Status Updated.vi"("error in (no error)"=w280, "Status"=w285, "Module ID"=w279) -> ("error out"=w286:errorcluster)  [unwired: 8 in]
          }
          frame "Connect" {
            w295 = "Connected to DB"  # Status
            # "Connect to database."
            n134 = call "Connect to DB.vi"("error in"=w302, "Data Cluster in"=w301) -> ("error out"=w296:errorcluster, "Data Cluster out"=w300:T2)  [unwired: 8 in]
            n135 = property on="Property Node" class="Mod Admin"(reference=w299) -> ("Accessors:Module ID"=w298:i32)  [unwired: 1 in, 2 out]
            n136 = call "Status Updated.vi"("error in (no error)"=w296, "Status"=w295, "Module ID"=w298) -> ("error out"=w297:errorcluster)  [unwired: 8 in]
          }
          frame "Query" {
            # "#debugging\nBC status or error"
            # "Send a SQL-Query to the database."
            n137 = Variant To Data(error in=w322, type=T11 {"Module ID"=-1, "Query"="", "Wait Notifier"=refnum, "wait for reply"=FALSE} ("Query Argument"), Variant=w321) -> (data=w320:T11, error out=w312:errorcluster)
            n138 = property on="Property Node" class="Mod Admin"(reference=w306) -> ("Accessors:Module ID"=w303:i32)  [unwired: 1 in, 2 out]
            n139 = Unbundle By Name(w314) -> ("DB-Interface"=w315:refnum<class "DB-Interface.lvclass">)
            n140 = Unbundle By Name(w320) -> ("Query"=w305:string, "Wait Notifier"=w319:refnum<notifier>)
            n141 = call-dynamic "Query.vi"("Query"=w305, "DB-Engine in"=w315) -> ("error out"=w311:errorcluster, "Meta Data"=w308:variant, "Return Data"=w309:string[][], "DB-Engine out"=w310:refnum<class "DB-Interface.lvclass">, "Field Names"=w307:string[])  [unwired: 5 in]
            n142 = case shown="Error" w311 {
              selector: w311 -> [_ w326]
              tunnel: w303 -> [w324 w327]
              tunnel: w305 -> [w323 w325]
              frame No Error {
                n143 = call "Status Updated.vi"("Status"=w323, "Module ID"=w324) -> ()  [unwired: 9 in, 1 out]
              }
              frame Error {
                n144 = call "Error Reported.vi"("Additional Information"=w325, "Error"=w326, "Module ID"=w327) -> ()  [unwired: 8 in, 1 out]
              }
            }
            n145 = flat-sequence {
              tunnel: w319 -> [w335]
              tunnel: [w335] -> w318
              tunnel: [w334] -> w317
              tunnel: w311 -> [w331]
              tunnel: w309 -> [w333]
              tunnel: w308 -> [w332]
              tunnel: w307 -> [w330]
              tunnel: w303 -> [w328]
              tunnel: w318 -> [w337]
              tunnel: w317 -> [w336]
              frame #0 {
                n146 = Bundle By Name(cluster=T18 {"Return Data"=[], "Meta Data"=variant, "Field Names"=[], "Query_error"={"status"=FALSE, "code"=0, "source"=""}, "Module ID"=0} ("Query (Reply Payload)"), "Return Data"=w333, "Meta Data"=w332, "Field Names"=w330, "Query_error"=w331, "Module ID"=w328) -> (w334:T18)
              }
              frame #1 {
                n147 = Send Notification(notification=w336, notifier=w337) -> ()  [unwired: 1 in, 2 out]
              }
            }
            n148 = Merge Errors(w312) -> (w316:errorcluster)
            n149 = Bundle By Name(cluster=w314, "DB-Interface"=w310) -> (w313:T2)
          }
          frame "Fast Query" {
            # "An asynchonous query to the DB. This request does not block and has no reply. To receive the db response register to the corresponding broadcast."
            n150 = Variant To Data(error in=w355, type=T7 {"Module ID"=-1, "Query"=""} ("Fast Query Argument"), Variant=w353) -> (data=w351:T7, error out=w354:errorcluster)
            n151 = Unbundle By Name(w343) -> ("DB-Interface"=w345:refnum<class "DB-Interface.lvclass">)
            n152 = property on="Property Node" class="Mod Admin"(reference=w341) -> ("Accessors:Module ID"=w340:i32)  [unwired: 1 in, 2 out]
            n153 = Unbundle By Name(w351) -> ("Query"=w344:string)
            n154 = call-dynamic "Query.vi"("Query"=w344, "DB-Engine in"=w345) -> ("error out"=w350:errorcluster, "Meta Data"=w347:variant, "Return Data"=w348:string[][], "DB-Engine out"=w349:refnum<class "DB-Interface.lvclass">, "Field Names"=w346:string[])  [unwired: 5 in]
            n155 = call "Fast Query Reply.vi"("Field Names"=w346, "error in (no error)"=w350, "Meta Data"=w347, "Return Data"=w348, "Module ID"=w340) -> ("error out"=w338:errorcluster)  [unwired: 6 in]
            n156 = Bundle By Name(cluster=w343, "DB-Interface"=w349) -> (w342:T2)
            n157 = Merge Errors(w354, w338) -> (w339:errorcluster)
          }
          frame "Start Transaction" {
            # "Start a transaction to get sure all following SQL commands get executed or none."
            n158 = Unbundle By Name(w359) -> ("DB-Interface"=w361:refnum<class "DB-Interface.lvclass">)
            n159 = call-dynamic "Start Transaction.vi"("error in"=w360, "DB-Interface in"=w361) -> ("error out"=w356:errorcluster, "DB-Interface out"=w357:refnum<class "DB-Interface.lvclass">)  [unwired: 8 in]
            n160 = Bundle By Name(cluster=w359, "DB-Interface"=w357) -> (w358:T2)
          }
          frame "Commit Transaction" {
            # "Commit a transaction. Either all SQL-commands get commited or, in case of an error, all get rejected."
            n161 = property class="Mod Admin"(reference=w362) -> ("Accessors:Module ID"=w363:i32)  [unwired: 1 in, 2 out]
            n162 = Variant To Data(error in=w375, type=T12 {"Module ID"=-1, "Wait Notifier"=refnum, "wait for reply"=FALSE} ("Commit Transaction Argument"), Variant=w374) -> (data=w373:T12, error out=w376:errorcluster)
            n163 = Unbundle By Name(w373) -> ("Wait Notifier"=w372:refnum<notifier>)
            n164 = Unbundle By Name(w367) -> ("DB-Interface"=w368:refnum<class "DB-Interface.lvclass">)
            n165 = call-dynamic "Commit Transaction.vi"("error in"=w376, "DB-Interface in"=w368) -> ("error out"=w377:errorcluster, "DB-Interface out"=w365:refnum<class "DB-Interface.lvclass">)  [unwired: 8 in]
            n166 = Bundle By Name(cluster=w367, "DB-Interface"=w365) -> (w366:T2)
            n167 = flat-sequence {
              tunnel: w372 -> [w382]
              tunnel: [w382] -> w371
              tunnel: [w381] -> w370
              tunnel: w377 -> [w380]
              tunnel: w363 -> [w378]
              tunnel: w371 -> [w384]
              tunnel: w370 -> [w383]
              frame #0 {
                n168 = Bundle By Name(cluster=T19 {"Commit Transaction_error"={"status"=FALSE, "code"=0, "source"=""}, "Module ID"=0} ("Commit Transaction (Reply Payload)"), "Commit Transaction_error"=w380, "Module ID"=w378) -> (w381:T19)
              }
              frame #1 {
                n169 = Send Notification(notification=w383, notifier=w384) -> ()  [unwired: 1 in, 2 out]
              }
            }
            n170 = Merge Errors(w376, w377) -> (w369:errorcluster)
          }
          frame "Rollback Transaction" {
            # "Rollback the active transaction."
            n171 = property class="Mod Admin"(reference=w385) -> ("Accessors:Module ID"=w386:i32)  [unwired: 1 in, 2 out]
            n172 = Variant To Data(error in=w400, type=T14 {"Module ID"=-1, "Wait Notifier"=refnum, "wait for reply"=FALSE} ("Rollback Transaction Argument"), Variant=w399) -> (data=w397:T14, error out=w401:errorcluster)
            n173 = Unbundle By Name(w397) -> ("Wait Notifier"=w396:refnum<notifier>, "wait for reply"=w395:bool)
            n174 = Unbundle By Name(w391) -> ("DB-Interface"=w390:refnum<class "DB-Interface.lvclass">)
            n175 = call-dynamic "Rollback Transaction.vi"("error in"=w401, "DB-Interface in"=w390) -> ("error out"=w387:errorcluster, "DB-Interface out"=w388:refnum<class "DB-Interface.lvclass">)  [unwired: 8 in]
            n176 = Merge Errors(w401, w387) -> (w392:errorcluster)
            n177 = Bundle By Name(cluster=w391, "DB-Interface"=w388) -> (w389:T2)
            n178 = Bundle By Name(cluster=T20 {"Rollback Transaction_error"={"status"=FALSE, "code"=0, "source"=""}, "Module ID"=0} ("Rollback Transaction (Reply Payload)"), "Rollback Transaction_error"=w387, "Module ID"=w386) -> (w394:T20)
            n179 = case shown="True" w395 {
              tunnel: w396 -> [_ w403]
              tunnel: w394 -> [_ w402]
              frame False {
              }
              frame True {
                n180 = Send Notification(notification=w402, notifier=w403) -> ()  [unwired: 1 in, 2 out]
              }
            }
          }
          frame "Close Connection" {
            # "Close connection to the database."
            n181 = Unbundle By Name(w411) -> ("DB-Interface"=w413:refnum<class "DB-Interface.lvclass">)
            n182 = property on="Property Node" class="Mod Admin"(reference=w407) -> ("Accessors:Module ID"=w405:i32)  [unwired: 1 in, 2 out]
            n183 = call-dynamic "Close.vi"("error in"=w412, "DB-Engine in"=w413) -> ("error out"=w408:errorcluster, "DB-Engine out"=w409:refnum<class "DB-Interface.lvclass">)  [unwired: 8 in]
            n184 = Bundle By Name(cluster=w411, "DB-Interface"=w409) -> (w410:T2)
            n185 = call "Status Updated.vi"("error in (no error)"=w408, "Status"="DB-connection closed", "Module ID"=w405) -> ("error out"=w406:errorcluster)  [unwired: 8 in]
          }
          frame "Get DB-Type" {
            # "Returns the type of the database in <b>DB-Type</b>"
            n186 = Variant To Data(error in=w425, type=T10 {"Module ID"=-1, "Wait Notifier"=refnum, "wait for reply"=FALSE} ("Get DB-Type Argument"), Variant=w423) -> (data=w421:T10, error out=w424:errorcluster)
            n187 = Unbundle By Name(w421) -> ("Wait Notifier"=w420:refnum<notifier>, "wait for reply"=w419:bool)
            n188 = Unbundle By Name(w418) -> ("DB-Interface"=w417:refnum<class "DB-Interface.lvclass">)
            n189 = call <vilib>:"Get LV Class Name.vi"("object"=w417) -> ("error out"=w415:errorcluster, "class name"=w416:string)  [unwired: 9 in]
            n190 = case shown="True" w419 {
              tunnel: w420 -> [_ w432]
              tunnel: w416 -> [_ w431]
              tunnel: w415 -> [_ w428]
              tunnel: w414 -> [_ w426]
              frame False {
              }
              frame True {
                n191 = property class="Mod Admin"(reference=w426) -> ("Accessors:Module ID"=w427:i32)  [unwired: 1 in, 2 out]
                n192 = Bundle By Name(cluster=T21 {"DB-Type"="", "error"={"status"=FALSE, "code"=0, "source"=""}, "Module ID"=0} ("Get DB-Type (Reply Payload)"), "DB-Type"=w431, "error"=w428, "Module ID"=w427) -> (w429:T21)
                n193 = Send Notification(notification=w429, notifier=w432) -> ()  [unwired: 1 in, 2 out]
              }
            }
          }
          frame "Set Module Timeout" {
            # "Overrides the DQMH internal Module Timeout with the specified value (must be greater than 0)"
            n194 = Variant To Data(error in=w444, type=T13 {"Module ID"=-1, "Module Timeout"=0} ("Set Module Timeout Argument"), Variant=w442) -> (data=w440:T13, error out=w437:errorcluster)
            n195 = Unbundle By Name(w440) -> ("Module Timeout"=w435:i32, "Module ID"=w434:i32)
            n196 = flat-sequence "Set the timeout and read it back to signal success \nor failure, in case the value is not greater than 0" {
              tunnel: w434 -> [w446]
              tunnel: w435 -> [w445]
              tunnel: w434 -> [w449]
              tunnel: [w448] -> w433
              frame #0 {
                n197 = call "timeout--fgv.vi"("Module ID"=w446, "Action"=timeout-fgv-actions--control."set", "Module Timeout in"=w445) -> ()  [unwired: 8 in, 1 out]
              }
              frame #1 {
                n198 = call "Module Timeout--constant.vi"("Module ID"=w449) -> ("Module Timeout"=w448:i32)  [unwired: 10 in]
              }
            }
            n199 = Format Into String(format string="set timeout to %d", w433) -> (resulting string=w438:string)  [unwired: 2 in, 1 out]
            n200 = call "Status Updated.vi"("error in (no error)"=w437, "Status"=w438, "Module ID"=w434) -> ("error out"=w436:errorcluster)  [unwired: 8 in]
          }
          frame "---Copy This Frame---" {
            # "Duplicate this frame when creating new messages.  Change this comment in the duplicated frame to describe this message."
            n201 = Merge Errors(w452) -> (w450:errorcluster)
          }
          frame "--- Exit and Error Handling---" {
            # "Separator - the following cases handle errors and exit messages."
          }
          frame "Error" {
            # "Error - Check the error message data and respond accordingly. This message is sent by the \"Error Handler\" VIs at the end of each loop in this application."
            n202 = property on="Property Node" class="Mod Admin"(reference=w460) -> ("Accessors:External Launch"=w457:bool, "Accessors:Module ID"=w459:i32)  [unwired: 1 in, 2 out]
            n203 = Variant To Data(error in=w465, type=errorcluster {"status"=FALSE, "code"=0, "source"=""} ("error constant"), Variant=w463) -> (data=w466:errorcluster, error out=w461:errorcluster)
            n204 = call "Error Reported.vi"("Error"=w466, "Module ID"=w459) -> ()  [unwired: 9 in, 1 out]
            n205 = case shown="False" w457 {
              tunnel: [w470 _] -> w458
              tunnel: w456 -> [w469 _]
              tunnel: w466 -> [_ _]
              frame False {
                # "If the module is running standalone, then pop up an error dialog and call the \"Exit\" message."
                n206 = call-poly <vilib>:"Delacor_lib_QMH_Enqueue Message (poly).vi"("Priority Message? (F)"=TRUE, "Message"="Exit", "Message Queue in"=w469) -> ("error out"=w470:errorcluster)  [unwired: 7 in, 1 out]
              }
              frame True {
                # "If the module was launched externally, calling the Error Reported broadcast VI is the only action performed by the \"Error\" message. The module's caller can then process the error appropriately."
              }
            }
            n207 = Merge Errors(w461, w458) -> (w455:errorcluster)
            n208 = local write "error out"(w455) -> ()
          }
          frame "Exit" {
            w487 = 91  # 91: not all Exit messages will have an argument
            w489 = TRUE  # Stop the VI
            # "Release the message queue reference"
            # "Exit - Exit the application."
            n209 = Variant To Data(error in=w490, type=T4 {"Origin"="", "Module ID"=-1, "Exit via Stop Module Req?"=FALSE, "Wait for Module to stop?"=FALSE} ("Stop Argument"), Variant=w485) -> (data=w482:T4, error out=w486:errorcluster)
            n210 = call <vilib>:"Clear Errors.vi"("error in (no error)"=w486, "specific error code to clear (0: all)"=w487) -> ("error out"=w477:errorcluster)  [unwired: 4 in, 1 out]
            n211 = control-ref of="This VI"() -> (w480:refnum<vi>)
            n212 = call "Handle Exit.vi"("Stop Argument"=w482, "Module Admin in"=w481, "VI reference"=w480) -> ("error out"=w472:errorcluster, "Wait for Stop?"=w483:bool)  [unwired: 7 in]
            n213 = Unbundle By Name(w474) -> ("DB-Interface"=w478:refnum<class "DB-Interface.lvclass">)
            n214 = call-dynamic "Close.vi"("DB-Engine in"=w478) -> ("DB-Engine out"=w475:refnum<class "DB-Interface.lvclass">)  [unwired: 9 in, 1 out]
            n215 = call-dynamic "Delacor_lib_QMH_Release Message Queue.vi"("error in"=w477, "Message Queue"=w476) -> ("error out"=w488:errorcluster)  [unwired: 9 in]
            n216 = Bundle By Name(cluster=w474, "DB-Interface"=w475) -> (w473:T2)
            n217 = property class="Mod Admin"(reference=w481) -> ("Accessors:Module ID"=w471:i32)  [unwired: 1 in, 2 out]
            n218 = Merge Errors(w488, w472) -> (w479:errorcluster)
            n219 = call "Error Reported.vi"("Error"=w479, "Module ID"=w471) -> ()  [unwired: 9 in, 1 out]
          }
          frame Default {
            # "'Default' case only runs if there is a message that isn't defined in any of the other cases.  Output a programming error."
            n220 = property on="Property Node" class="Mod Admin"(reference=w494) -> ("Accessors:Module ID"=w493:i32)  [unwired: 1 in, 2 out]
            n221 = call "Module Name--constant.vi"("Module ID"=w493) -> ("Module Name"=w495:string)  [unwired: 10 in]
            n222 = xnode "Error Ring"("parameter 0"=w496, "parameter 1"=w495) -> ("error out"=w497:errorcluster)
            n223 = Merge Errors(w491, w497) -> (w492:errorcluster)
          }
        }
        n224 = call-dynamic "Delacor_lib_QMH_Error Handler - Message Handling Loop.vi"("error in"=w239, "Message Queue in"=w230) -> ("dup error in"=w229:errorcluster)  [unwired: 8 in, 1 out]
      }
    }
    frame Error {
      n225 = call "Synchronize Caller Events.vi"("Module Admin"=w510) -> ("Module Admin out"=w509:refnum<class "Delacor_lib_QMH_Cloneable Module Admin.lvclass">)  [unwired: 9 in, 1 out]
      n226 = property on="Property Node" class="Mod Admin"(reference=w509) -> ("Accessors:Module ID"=w508:i32)  [unwired: 1 in, 2 out]
      n227 = call-dynamic "Delacor_lib_QMH_Release Message Queue.vi"("Message Queue"=w507) -> ()  [unwired: 10 in, 1 out]
      n228 = call "Module Name--constant.vi"("Module ID"=w508) -> ("Module Name"=w513:string)  [unwired: 10 in]
      n229 = Format Into String(format string="An error occurred during initialization. %s is no longer running.", w513) -> (resulting string=w511:string)  [unwired: 2 in, 1 out]
      n230 = call "Error Reported.vi"("Additional Information"=w511, "Error"=w514, "Module ID"=w508) -> ()  [unwired: 8 in, 1 out]
    }
  }
  n231 = Merge Errors(w17, w16) -> (w18:errorcluster)
  n232 = call "Close Module.vi"("error in (no error)"=w18, "Wait for stop?"=w7, "Module Admin in"=w8) -> ("error out"=w10:errorcluster, "External Launch"=w6:bool, "Module Admin out"=w1:refnum<class "Delacor_lib_QMH_Cloneable Module Admin.lvclass">)  [unwired: 6 in]
  n233 = Unregister For Events(event registration refnum=w14, error in=w10) -> (error out=w2:errorcluster)
  "error out" <- w2
  n234 = local write "Module Admin"(w1) -> ()
  n235 = case "External Launch?" shown="True" w6 {
    tunnel: w2 -> [_ w516]
    frame False {
    }
    frame True {
      n236 = case shown="No Error" w516 {
        frame No Error {
          n237 = invoke on="Invoke Node" class="VI" method="FP.Close"() -> ()  [unwired: 3 in, 3 out]
        }
        frame Error {
          n238 = invoke on="Invoke Node" class="VI" method="FP.Open"("Activate"=TRUE ("Activate?")) -> ()  [unwired: 4 in, 5 out]
        }
      }
    }
  }
